vi "Remove Channel.vi"(7 "name":string, 8 "error in (no error)":errorcluster, 11 "refnum":T1) -> (0 "error out":errorcluster, 2 "exists?":bool, 3 "refnum out":T1)   [LabVIEW 2017, in "DSF Configuration API.lvlib"]
doc: "Removes a section from the configuration data identified by <B>refnum</B>."
uses:
  DSF Configuration API.lvlib
  Controls/DSF Config Data RefNum.ctl
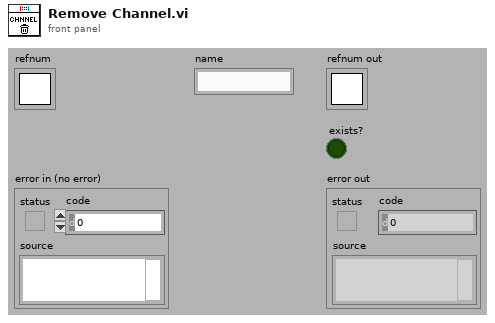
[diagram p1: front panel]
types:
  T1 = typedef "DSF Configuration API.lvlib/DSF Config Data RefNum.ctl" = refnum<k1>
  T2 = typedef "DSF Configuration API.lvlib/Config Queue.ctl" = refnum<queue>
  T3 = typedef "DSF Configuration API.lvlib/Config Data.ctl" = cluster{"dsf configuration":T4, "path":path, "dirty":bool}
  T4 = typedef "DSF Configuration API.lvlib/DSF Config.ctl" = cluster{"dsfversion":T5, "version":T5, "plugins":T6[], "groups":T9[], "transfers":T11[], "channels":T13[], "settings":T15[]}
  T5 = typedef "DSF Configuration API.lvlib/Version Info.ctl" = cluster{"major":u32, "minor":u32, "fix":u32, "build":string}
  T6 = typedef "DSF Configuration API.lvlib/DSF Plugin.ctl" = cluster{"id":string, "values":T7}
  T7 = typedef "DSF Configuration API.lvlib/DSF Plugin Info.ctl" = cluster{"type":string, "timing":T8, "group ids":string[], "settings id":string}
  T8 = typedef "DSF Configuration API.lvlib/DSF Timing Info.ctl" = cluster{"decimation":i32, "offset":i32}
  T9 = typedef "DSF Configuration API.lvlib/DSF Group.ctl" = cluster{"id":string, "values":T10}
  T10 = typedef "DSF Configuration API.lvlib/DSF Group Info.ctl" = cluster{"direction":i32, "timing":T8, "transfer ids":string[], "settings id":string}
  T11 = typedef "DSF Configuration API.lvlib/DSF Transfer.ctl" = cluster{"id":string, "values":T12}
  T12 = typedef "DSF Configuration API.lvlib/DSF Transfer Info.ctl" = cluster{"byte order":i32, "channel ids":string[], "settings id":string}
  T13 = typedef "DSF Configuration API.lvlib/DSF Channel.ctl" = cluster{"id":string, "values":T14}
  T14 = typedef "DSF Configuration API.lvlib/DSF Channel Info.ctl" = cluster{"count":i32, "offset":i32, "data type":i32, "resource path":string, "settings id":string}
  T15 = typedef "DSF Configuration API.lvlib/DSF Settings.ctl" = cluster{"id":string, "values":T16}
  T16 = typedef "DSF Configuration API.lvlib/DSF Settings Info.ctl" = cluster{"key":string, "value":string}[]
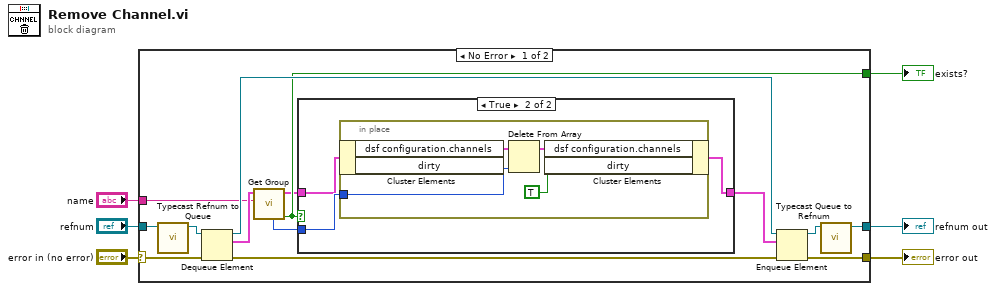
[diagram p0: block diagram]
diagram:
  n1 = case shown="No Error" "error in (no error)" {
    selector: "error in (no error)" -> [w12 w30]
    tunnel: [w17 w30] -> w1
    tunnel: [w14 w29] -> w3
    tunnel: "refnum" -> [w16 w29]
    tunnel: "name" -> [w10 _]
    tunnel: [w9 _] -> w2
    frame No Error {
      n2 = call "Typecast Refnum to Queue.vi"("refnum in"=w16) -> ("queue out"=w13:T2)  [unwired: 10 out]
      n3 = Dequeue Element(queue=w13, error in (no error)=w12) -> (queue out=w19:T2, element=w11:T3, error out=w18:errorcluster)  [unwired: 2 out]
      n4 = call "Get Group.vi"("id"=w10, "element"=w11) -> ("exists?"=w9:bool, "element out"=w8:T3, "index"=w7:i32)  [unwired: 6 in, 1 out]
      n5 = case shown="True" w9 {
        tunnel: [w21 w24] -> w20
        tunnel: w7 -> [_ w23]
        tunnel: w8 -> [w21 w22]
        frame False {
        }
        frame True {
          n6 = in-place {
            in-place-border: w23 -> [w28]
            n7 = in-place-cluster #1(w22) -> ("dsf configuration.channels"=w27:T13[])  [unwired: 1 out]
            n8 = Delete From Array(array=w27, index=w28) -> (array with subset deleted=w26:T13[])  [unwired: 1 in, 1 out]
            n9 = in-place-cluster #1("dsf configuration.channels"=w26, "dirty"=TRUE) -> (w24:T3)
          }
        }
      }
      n10 = Enqueue Element(queue=w19, element=w20, error in (no error)=w18) -> (queue out=w15:T2, error out=w17:errorcluster)  [unwired: 2 out]
      n11 = call "Typecast Queue to Refnum.vi"("queue in"=w15) -> ("refnum out"=w14:T1)  [unwired: 10 out]
    }
    frame Error {
    }
  }
  "error out" <- w1
  "exists?" <- w2
  "refnum out" <- w3
